vi "FTW-CodeGen-Prototype.vi"(0 "REPLACED_Connection":refnum<k24>, 2 "REPLACED_SQL Script":string, 5 "ADAPT_Row Datatype":cluster{"Column":variant}, 11 "REPLACED_error in":errorcluster) -> (4 "REPLACED_Connection out":refnum<k24>, 6 "ADAPT_Result Set":cluster{"Column":variant}[](array[cluster]), 8 "REPLACED_Time to Execute":dbl format="%.6fsec", 15 "REPLACED_error out":errorcluster)   [LabVIEW 2015, in "FTW-dotNet-SQL-Fetch.xnode"]
uses:
  FTW-dotNet-SQL-Fetch.xnode
  System.Data
  src/error/FTW-ERR-ThrowError.vi
  src/error/FTW-ERR-StatusException.vi
  src/error/FTW-ERR-CallChain.vi
  src/string/FTW-STR-ReplaceWhitespace.vi
  src/string/FTW-STR-Array-Delimit.vi
  src/error/FTW-ERR-Clear.vi
  src/regex/FTW-Regex-ReplaceAll.vi
panel:
  # "Inputs"
  # "Outputs"
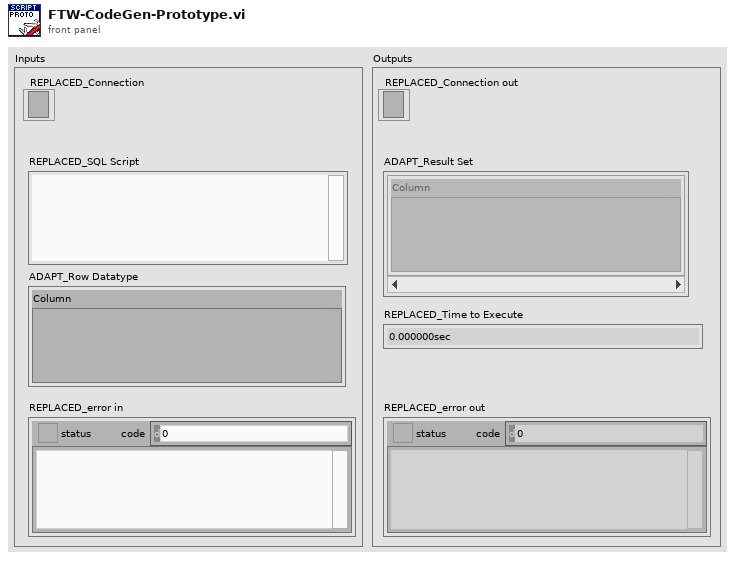
[diagram p1: front panel]
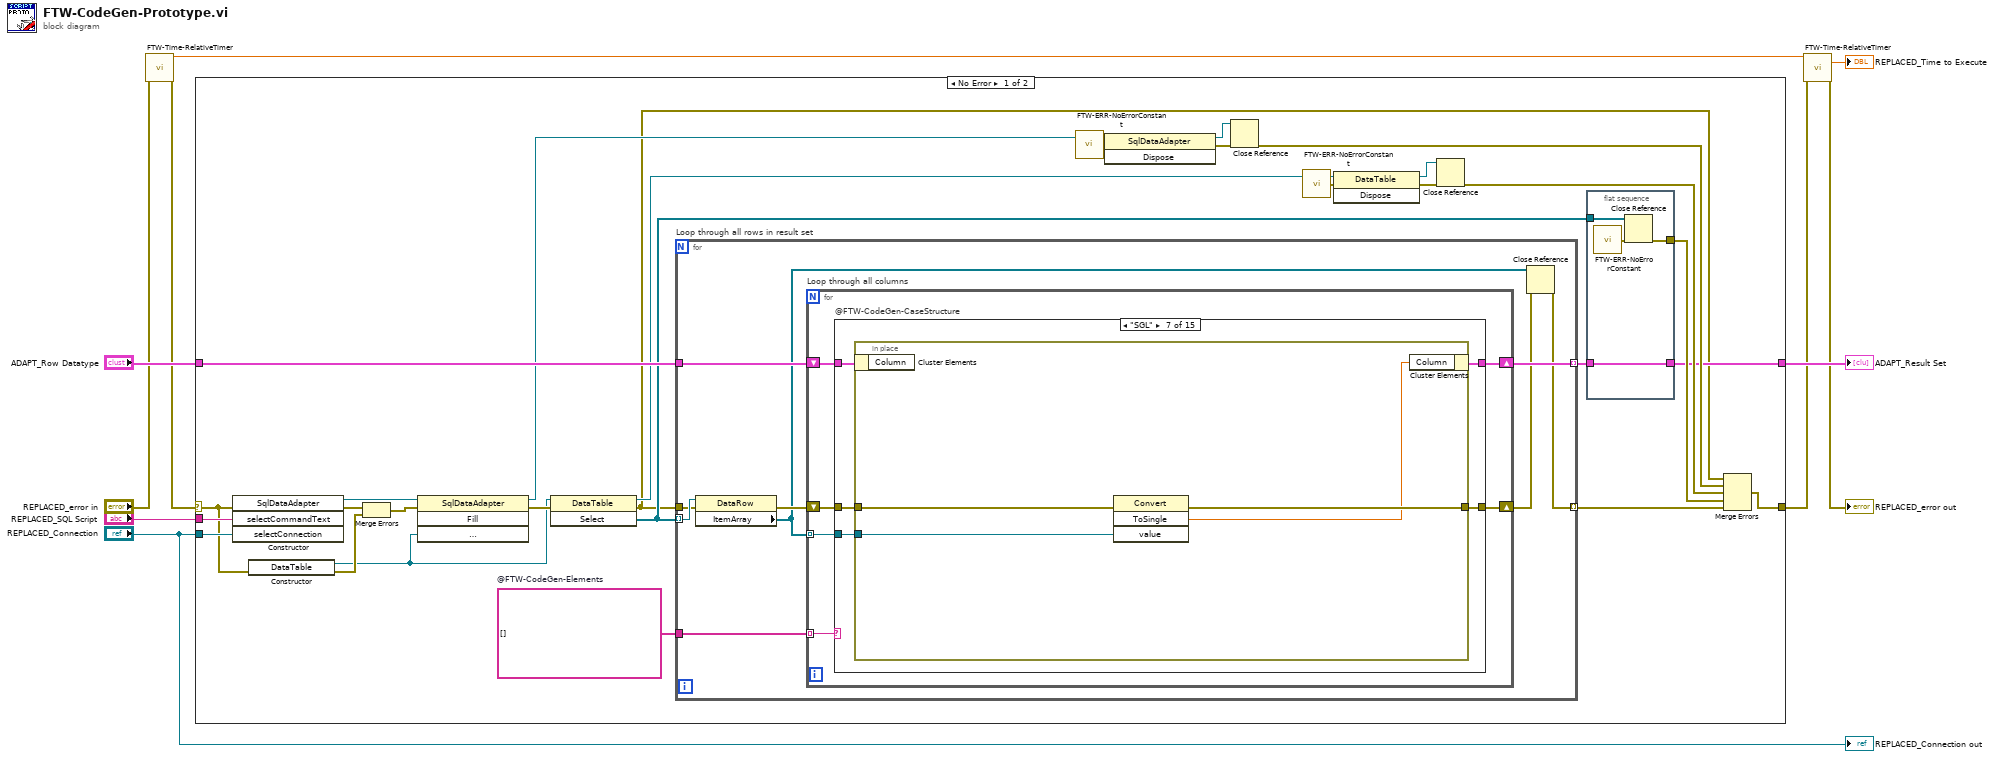
[diagram p0: block diagram]
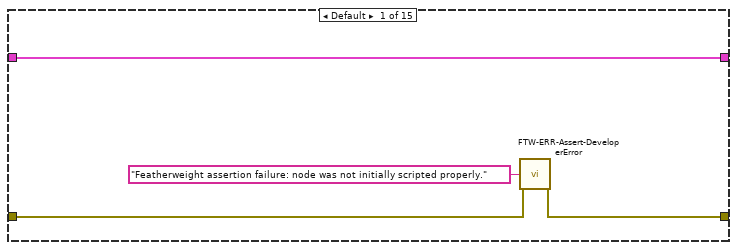
[diagram p2: hidden frame]
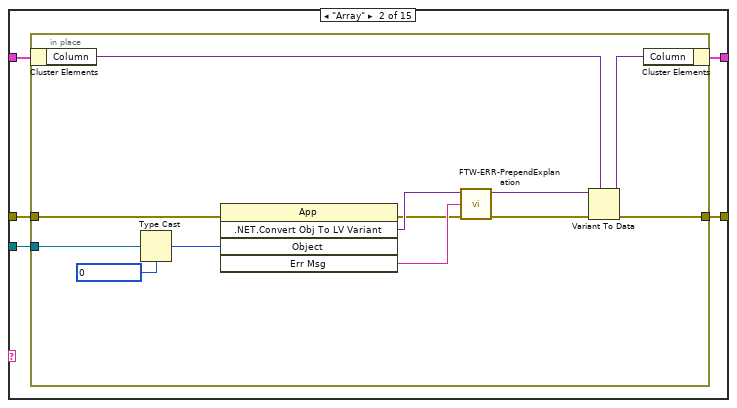
[diagram p3: hidden frame]
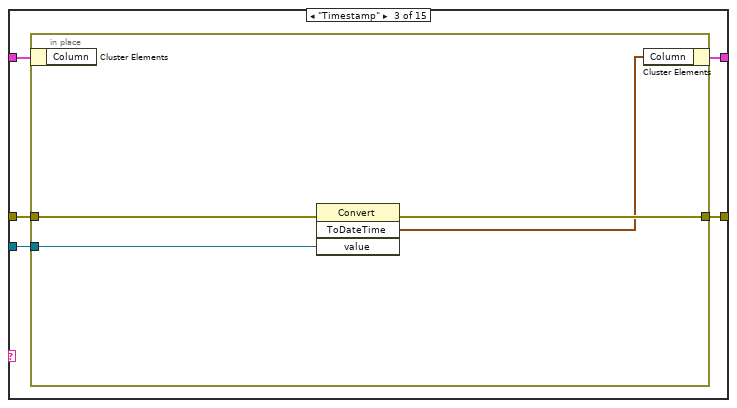
[diagram p4: hidden frame]
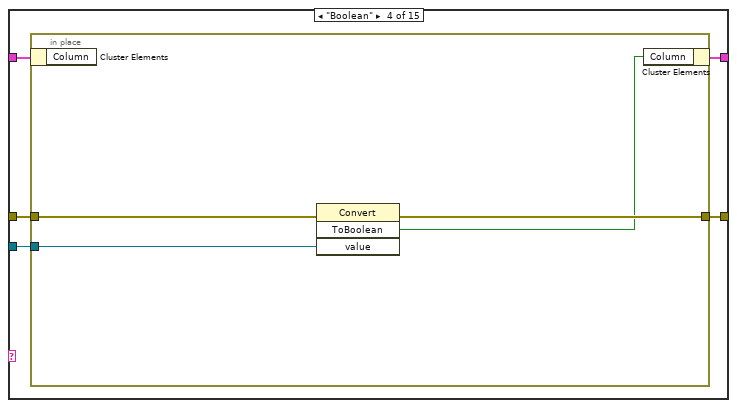
[diagram p5: hidden frame]
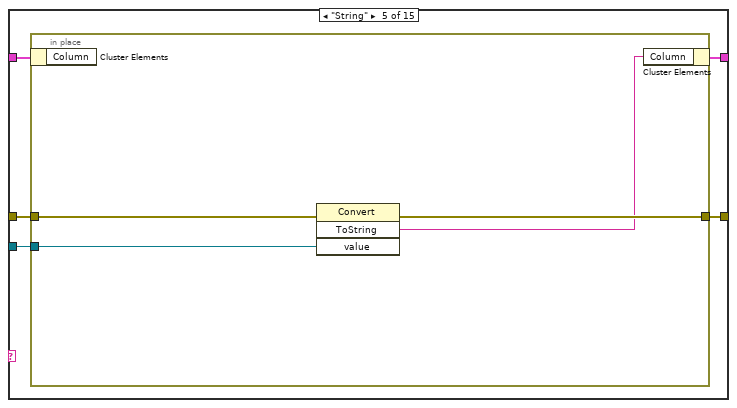
[diagram p6: hidden frame]
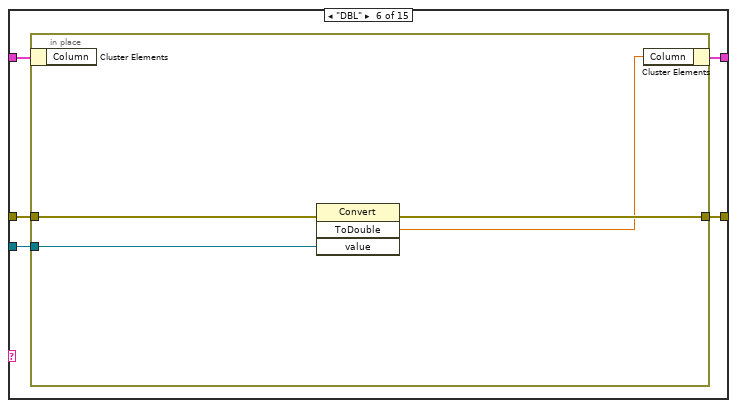
[diagram p7: hidden frame]
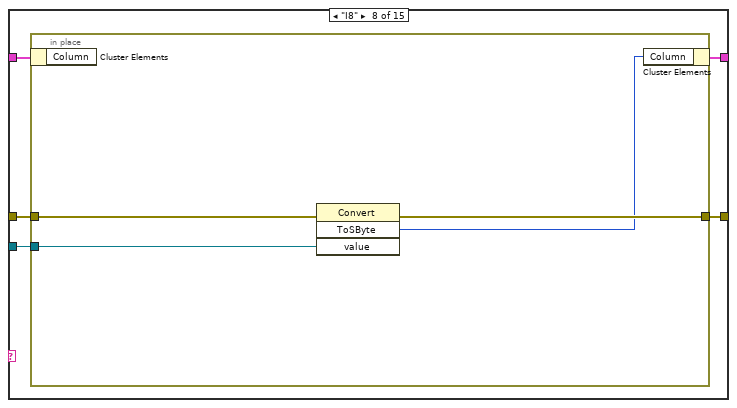
[diagram p8: hidden frame]
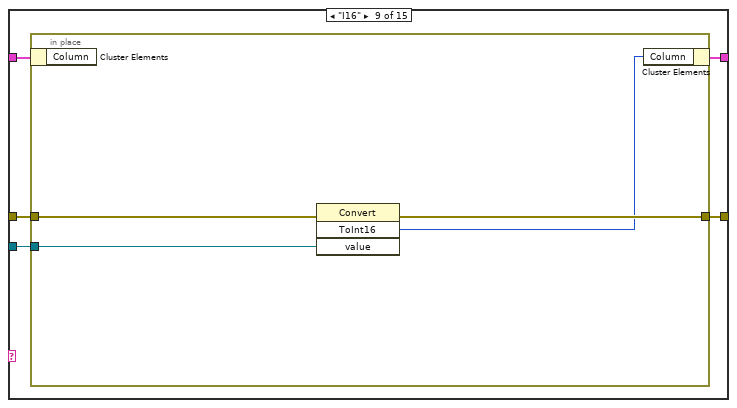
[diagram p9: hidden frame]
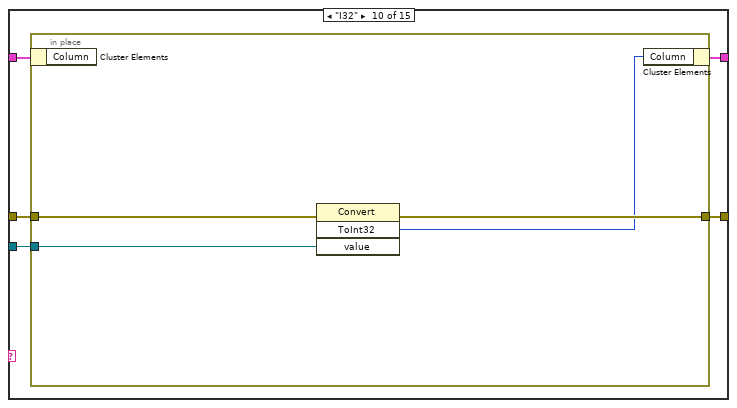
[diagram p10: hidden frame]
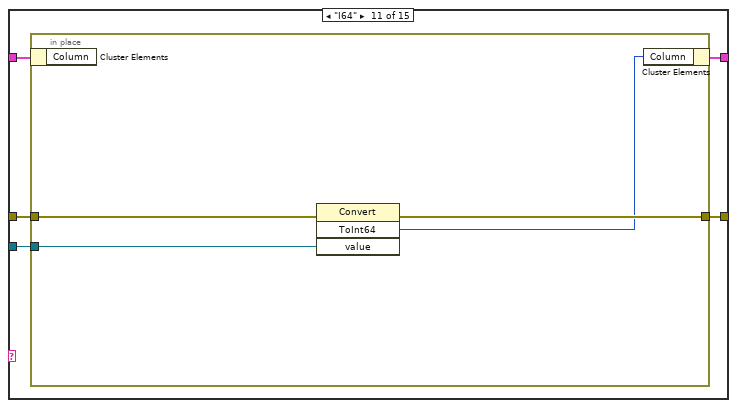
[diagram p11: hidden frame]
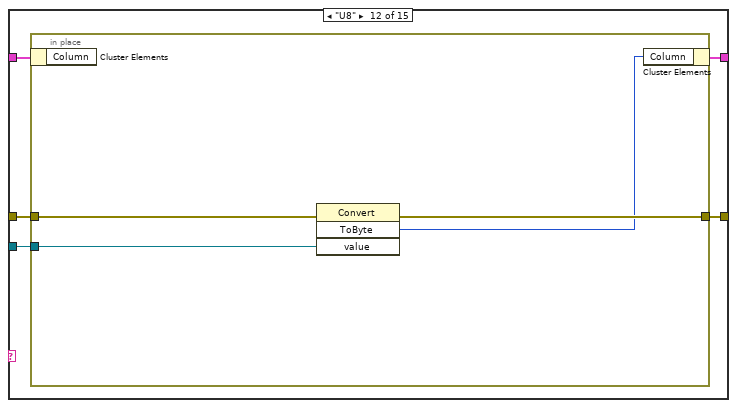
[diagram p12: hidden frame]
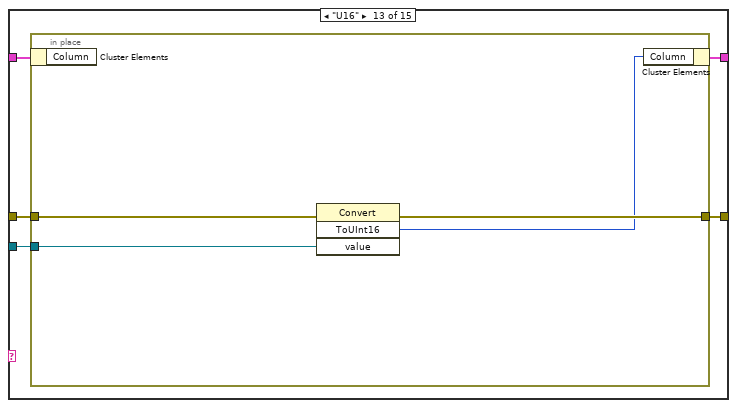
[diagram p13: hidden frame]
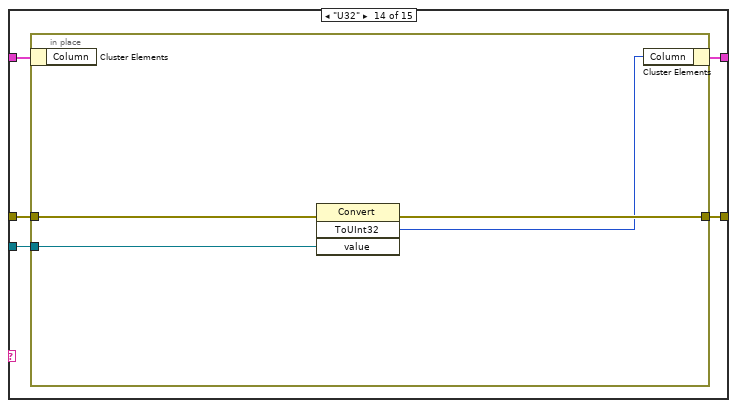
[diagram p14: hidden frame]
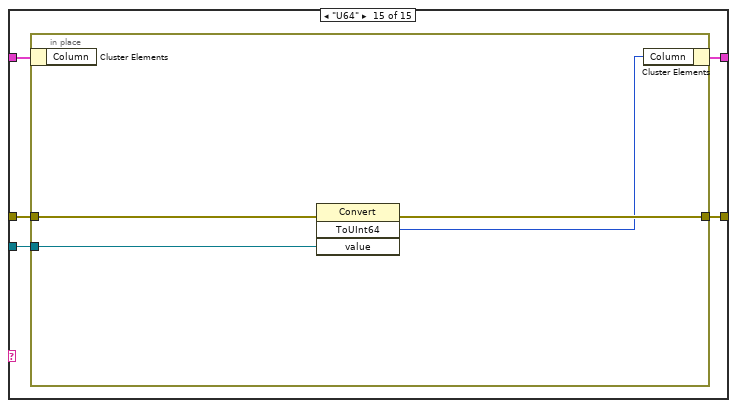
[diagram p15: hidden frame]
diagram:
  n1 = call "FTW-Time-RelativeTimer.vi"("error in"="REPLACED_error in") -> ("Current Timer Value"=w4:dbl, "error out"=w7:errorcluster)  [unwired: 12 in, 1 out]
  n2 = case shown="No Error" w7 {
    selector: w7 -> [w16 w195]
    tunnel: "REPLACED_SQL Script" -> [w17 _]
    tunnel: [w18 w195] -> w5
    tunnel: "ADAPT_Row Datatype" -> [w38 _]
    tunnel: [w19 _] -> w8
    tunnel: "REPLACED_Connection" -> [w22 _]
    frame No Error {
      w13 = string[] []  # @FTW-CodeGen-Elements
      n3 = constructor class="SqlDataAdapter"(error in=w16, "selectCommandText"=w17, "selectConnection"=w22) -> (reference out=w37:refnum<k24>, error out=w34:errorcluster)  [unwired: 2 in, 3 out]
      n4 = constructor class="DataTable"(error in=w16) -> (reference out=w26:refnum<k24>, error out=w32:errorcluster)  [unwired: 2 in, 1 out]
      n5 = Merge Errors(w34, w32) -> (w33:errorcluster)
      n6 = invoke class="SqlDataAdapter" method="Fill"(reference=w37, error in=w33, "dataTable"=w26) -> (reference out=w29:refnum<k24>, error out=w28:errorcluster)  [unwired: 1 in, 2 out]
      n7 = invoke class="DataTable" method="Select"(reference=w26, error in=w28) -> (reference out=w25:refnum<k24>, error out=w11:errorcluster, "Select"=w12:refnum<k24>[])  [unwired: 1 in]
      n8 = for "Loop through all rows in result set" {
        tunnel: w38 -> [w50]
        tunnel: [w51] -> w15 mode=indexing
        tunnel: w12 -> [w49] mode=indexing
        tunnel: w11 -> [w48]
        tunnel: [w47] -> w14 mode=indexing
        tunnel: w13 -> [w46]
        n9 = property class="DataRow"(reference=w49, error in=w48) -> (error out=w45:errorcluster, "ItemArray"=w44:refnum<k24>[])  [unwired: 1 out]
        n10 = for "Loop through all columns" {
          shift-right: [w57] -> w43
          shift-left: w45 -> [w53]
          shift-right: [w55] -> w51
          shift-left: w50 -> [w56]
          tunnel: w46 -> [w54] mode=indexing
          tunnel: w44 -> [w52] mode=indexing
          n11 = case "@FTW-CodeGen-CaseStructure" shown="\"SGL\"" w54 {
            tunnel: w53 -> [w60 w65 w81 w90 w99 w108 w117 w126 w135 w144 w153 w162 w171 w180 w189]
            tunnel: [w59 w66 w82 w91 w100 w109 w118 w127 w136 w145 w154 w163 w172 w181 w190] -> w57
            tunnel: w56 -> [w61 w63 w79 w88 w97 w106 w115 w124 w133 w142 w151 w160 w169 w178 w187]
            tunnel: [w61 w62 w78 w87 w96 w105 w114 w123 w132 w141 w150 w159 w168 w177 w186] -> w55
            tunnel: w52 -> [_ w64 w80 w89 w98 w107 w116 w125 w134 w143 w152 w161 w170 w179 w188]
            frame Default {
              n12 = call "FTW-ERR-Assert-DeveloperError.vi"("Reason this error should never happen"="Featherweight assertion failure: node was not initially scripted properly.", "error in"=w60) -> ("error out"=w59:errorcluster)  [unwired: 13 in]
            }
            frame "Array" {
              n13 = in-place "In Place Element Structure" {
                in-place-border: [w75] -> w66
                in-place-border: w65 -> [w71]
                in-place-border: w64 -> [w74]
                n14 = in-place-cluster #1 ("Unbundle / Bundle Elements")(w63) -> ("Column"=w77:variant)
                n15 = Type Cast(type=u32 0, x=w74) -> (*(type *) &x=w73:u32)
                n16 = invoke class="App" method=".NET.Convert Obj To LV Variant"(error in=w71, "Object"=w73) -> (error out=w68:errorcluster, "Convert .NET Object To LV Variant"=w72:variant, "Err Msg"=w69:string)  [unwired: 3 in, 2 out]
                n17 = call "FTW-ERR-PrependExplanation.vi"("Exception Information"=w69, "error in"=w68) -> ("error out"=w67:errorcluster)  [unwired: 13 in]
                n18 = Variant To Data(error in=w67, type=w77, Variant=w72) -> (data=w76:variant, error out=w75:errorcluster)
                n19 = in-place-cluster #1 ("Unbundle / Bundle Elements")("Column"=w76) -> (w62:cluster{"Column":variant})
              }
            }
            frame "Timestamp" {
              n20 = in-place "In Place Element Structure" {
                in-place-border: [w85] -> w82
                in-place-border: w81 -> [w86]
                in-place-border: w80 -> [w83]
                n21 = in-place-cluster #2 ("Unbundle / Bundle Elements")(w79) -> ()  [unwired: 1 out]
                n22 = invoke class="Convert" method="ToDateTime"(error in=w86, "value"=w83) -> (error out=w85:errorcluster, "ToDateTime"=w84:timestamp)  [unwired: 2 in, 2 out]
                n23 = in-place-cluster #2 ("Unbundle / Bundle Elements")("Column"=w84) -> (w78:cluster{"Column":variant})
              }
            }
            frame "Boolean" {
              n24 = in-place "In Place Element Structure" {
                in-place-border: [w94] -> w91
                in-place-border: w90 -> [w95]
                in-place-border: w89 -> [w92]
                n25 = in-place-cluster #3 ("Unbundle / Bundle Elements")(w88) -> ()  [unwired: 1 out]
                n26 = invoke class="Convert" method="ToBoolean"(error in=w95, "value"=w92) -> (error out=w94:errorcluster, "ToBoolean"=w93:bool)  [unwired: 2 in, 2 out]
                n27 = in-place-cluster #3 ("Unbundle / Bundle Elements")("Column"=w93) -> (w87:cluster{"Column":variant})
              }
            }
            frame "String" {
              n28 = in-place "In Place Element Structure" {
                in-place-border: [w103] -> w100
                in-place-border: w99 -> [w104]
                in-place-border: w98 -> [w101]
                n29 = in-place-cluster #4 ("Unbundle / Bundle Elements")(w97) -> ()  [unwired: 1 out]
                n30 = invoke class="Convert" method="ToString"(error in=w104, "value"=w101) -> (error out=w103:errorcluster, "ToString"=w102:string)  [unwired: 2 in, 2 out]
                n31 = in-place-cluster #4 ("Unbundle / Bundle Elements")("Column"=w102) -> (w96:cluster{"Column":variant})
              }
            }
            frame "DBL" {
              n32 = in-place "In Place Element Structure" {
                in-place-border: [w112] -> w109
                in-place-border: w108 -> [w113]
                in-place-border: w107 -> [w110]
                n33 = in-place-cluster #5 ("Unbundle / Bundle Elements")(w106) -> ()  [unwired: 1 out]
                n34 = invoke class="Convert" method="ToDouble"(error in=w113, "value"=w110) -> (error out=w112:errorcluster, "ToDouble"=w111:dbl)  [unwired: 2 in, 2 out]
                n35 = in-place-cluster #5 ("Unbundle / Bundle Elements")("Column"=w111) -> (w105:cluster{"Column":variant})
              }
            }
            frame "SGL" {
              n36 = in-place "In Place Element Structure" {
                in-place-border: [w121] -> w118
                in-place-border: w117 -> [w122]
                in-place-border: w116 -> [w119]
                n37 = in-place-cluster #6 ("Unbundle / Bundle Elements")(w115) -> ()  [unwired: 1 out]
                n38 = invoke class="Convert" method="ToSingle"(error in=w122, "value"=w119) -> (error out=w121:errorcluster, "ToSingle"=w120:sgl)  [unwired: 2 in, 2 out]
                n39 = in-place-cluster #6 ("Unbundle / Bundle Elements")("Column"=w120) -> (w114:cluster{"Column":variant})
              }
            }
            frame "I8" {
              n40 = in-place "In Place Element Structure" {
                in-place-border: [w130] -> w127
                in-place-border: w126 -> [w131]
                in-place-border: w125 -> [w128]
                n41 = in-place-cluster #7 ("Unbundle / Bundle Elements")(w124) -> ()  [unwired: 1 out]
                n42 = invoke class="Convert" method="ToSByte"(error in=w131, "value"=w128) -> (error out=w130:errorcluster, "ToSByte"=w129:i8)  [unwired: 2 in, 2 out]
                n43 = in-place-cluster #7 ("Unbundle / Bundle Elements")("Column"=w129) -> (w123:cluster{"Column":variant})
              }
            }
            frame "I16" {
              n44 = in-place "In Place Element Structure" {
                in-place-border: [w139] -> w136
                in-place-border: w135 -> [w140]
                in-place-border: w134 -> [w137]
                n45 = in-place-cluster #8 ("Unbundle / Bundle Elements")(w133) -> ()  [unwired: 1 out]
                n46 = invoke class="Convert" method="ToInt16"(error in=w140, "value"=w137) -> (error out=w139:errorcluster, "ToInt16"=w138:i16)  [unwired: 2 in, 2 out]
                n47 = in-place-cluster #8 ("Unbundle / Bundle Elements")("Column"=w138) -> (w132:cluster{"Column":variant})
              }
            }
            frame "I32" {
              n48 = in-place "In Place Element Structure" {
                in-place-border: [w148] -> w145
                in-place-border: w144 -> [w149]
                in-place-border: w143 -> [w146]
                n49 = in-place-cluster #9 ("Unbundle / Bundle Elements")(w142) -> ()  [unwired: 1 out]
                n50 = invoke class="Convert" method="ToInt32"(error in=w149, "value"=w146) -> (error out=w148:errorcluster, "ToInt32"=w147:i32)  [unwired: 2 in, 2 out]
                n51 = in-place-cluster #9 ("Unbundle / Bundle Elements")("Column"=w147) -> (w141:cluster{"Column":variant})
              }
            }
            frame "I64" {
              n52 = in-place "In Place Element Structure" {
                in-place-border: [w157] -> w154
                in-place-border: w153 -> [w158]
                in-place-border: w152 -> [w155]
                n53 = in-place-cluster #10 ("Unbundle / Bundle Elements")(w151) -> ()  [unwired: 1 out]
                n54 = invoke class="Convert" method="ToInt64"(error in=w158, "value"=w155) -> (error out=w157:errorcluster, "ToInt64"=w156:i64)  [unwired: 2 in, 2 out]
                n55 = in-place-cluster #10 ("Unbundle / Bundle Elements")("Column"=w156) -> (w150:cluster{"Column":variant})
              }
            }
            frame "U8" {
              n56 = in-place "In Place Element Structure" {
                in-place-border: [w166] -> w163
                in-place-border: w162 -> [w167]
                in-place-border: w161 -> [w164]
                n57 = in-place-cluster #11 ("Unbundle / Bundle Elements")(w160) -> ()  [unwired: 1 out]
                n58 = invoke class="Convert" method="ToByte"(error in=w167, "value"=w164) -> (error out=w166:errorcluster, "ToByte"=w165:u8)  [unwired: 2 in, 2 out]
                n59 = in-place-cluster #11 ("Unbundle / Bundle Elements")("Column"=w165) -> (w159:cluster{"Column":variant})
              }
            }
            frame "U16" {
              n60 = in-place "In Place Element Structure" {
                in-place-border: [w175] -> w172
                in-place-border: w171 -> [w176]
                in-place-border: w170 -> [w173]
                n61 = in-place-cluster #12 ("Unbundle / Bundle Elements")(w169) -> ()  [unwired: 1 out]
                n62 = invoke class="Convert" method="ToUInt16"(error in=w176, "value"=w173) -> (error out=w175:errorcluster, "ToUInt16"=w174:u16)  [unwired: 2 in, 2 out]
                n63 = in-place-cluster #12 ("Unbundle / Bundle Elements")("Column"=w174) -> (w168:cluster{"Column":variant})
              }
            }
            frame "U32" {
              n64 = in-place "In Place Element Structure" {
                in-place-border: [w184] -> w181
                in-place-border: w180 -> [w185]
                in-place-border: w179 -> [w182]
                n65 = in-place-cluster #13 ("Unbundle / Bundle Elements")(w178) -> ()  [unwired: 1 out]
                n66 = invoke class="Convert" method="ToUInt32"(error in=w185, "value"=w182) -> (error out=w184:errorcluster, "ToUInt32"=w183:u32)  [unwired: 2 in, 2 out]
                n67 = in-place-cluster #13 ("Unbundle / Bundle Elements")("Column"=w183) -> (w177:cluster{"Column":variant})
              }
            }
            frame "U64" {
              n68 = in-place "In Place Element Structure" {
                in-place-border: [w193] -> w190
                in-place-border: w189 -> [w194]
                in-place-border: w188 -> [w191]
                n69 = in-place-cluster #14 ("Unbundle / Bundle Elements")(w187) -> ()  [unwired: 1 out]
                n70 = invoke class="Convert" method="ToUInt64"(error in=w194, "value"=w191) -> (error out=w193:errorcluster, "ToUInt64"=w192:u64)  [unwired: 2 in, 2 out]
                n71 = in-place-cluster #14 ("Unbundle / Bundle Elements")("Column"=w192) -> (w186:cluster{"Column":variant})
              }
            }
          }
        }
        n72 = Close Reference(reference=w44, error in (no error)=w43) -> (error out=w47:errorcluster)
      }
      n73 = call "FTW-ERR-NoErrorConstant.vi"() -> ("no error"=w23:errorcluster)
      n74 = invoke class="SqlDataAdapter" method="Dispose"(reference=w29, error in=w23) -> (reference out=w31:refnum<k24>, error out=w30:errorcluster)  [unwired: 1 in, 1 out]
      n75 = Close Reference(reference=w31, error in (no error)=w30) -> (error out=w20:errorcluster)
      n76 = call "FTW-ERR-NoErrorConstant.vi"() -> ("no error"=w24:errorcluster)
      n77 = invoke class="DataTable" method="Dispose"(reference=w25, error in=w24) -> (reference out=w35:refnum<k24>, error out=w36:errorcluster)  [unwired: 1 in, 1 out]
      n78 = Close Reference(reference=w35, error in (no error)=w36) -> (error out=w27:errorcluster)
      n79 = flat-sequence {
        tunnel: w12 -> [w42]
        tunnel: [w41] -> w19
        tunnel: w15 -> [w41]
        tunnel: [w39] -> w21
        frame #0 {
          n80 = call "FTW-ERR-NoErrorConstant.vi"() -> ("no error"=w40:errorcluster)
          n81 = Close Reference(reference=w42, error in (no error)=w40) -> (error out=w39:errorcluster)
        }
      }
      n82 = Merge Errors(w11, w20, w27, w21, w14) -> (w18:errorcluster)
    }
    frame Error {
    }
  }
  "ADAPT_Result Set" <- w8
  n83 = call "FTW-Time-RelativeTimer.vi"("Previous Timer Value"=w4, "error in"=w5) -> ("Elapsed Time"=→"REPLACED_Time to Execute":dbl, "error out"=→"REPLACED_error out":errorcluster)  [unwired: 11 in, 1 out]
  "REPLACED_Connection out" <- "REPLACED_Connection"
